vi "Generate Request ID.vi"() -> (3 "Generate Request ID":u32)   [LabVIEW 2020, in "WAMP Client.lvclass"]
uses:
  <userlib>/lvwamp/WAMP Client/WAMP Client.lvclass
  <vilib>/numeric/Random Number (Range) U64.vi
  <vilib>/numeric/sub_Random U32.vi
  <userlib>/lvwamp/WAMP Client/WAMP Client.lvclass/WAMP Client.ctl
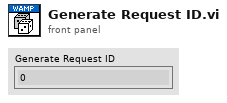
[diagram p1: front panel]
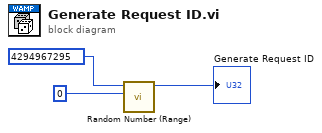
[diagram p0: block diagram]
diagram:
  n1 = call-poly <vilib>:"Random Number (Range).vi"("lower bound (0)"=u32 0, "upper bound (100)"=u32 4294967295) -> ("number"=→"Generate Request ID":u64)  [unwired: 9 in]
